vi "data_output_continuous.vi"() -> ()   [LabVIEW 2017]
uses:
  <vilib>/Utility/error.llb/DialogType.ctl
  <vilib>/DAQmx/write.llb/DAQmx Write (Analog 1D Wfm NChan NSamp).vi
  <vilib>/Utility/file.llb/Read Delimited Spreadsheet (DBL).vi
  <vilib>/DAQmx/create/channels.llb/DAQmx Create Channel (AO-Voltage-Basic).vi
  <vilib>/DAQmx/configure/timing.llb/DAQmx Timing (Sample Clock).vi
  <vilib>/DAQmx/miscellaneous.llb/DAQmx Fill In Error Info.vi
panel:
  in  "OK Button":bool
  out "Amplitude":dbl
  in  "Reduce Amplitude":bool
  in  "Sample Rate":dbl=1000.0
  in  "Sample Clock Source":tag="OnboardClock"
  in  "Max Voltage":dbl=5.0
  in  "Min Voltage":dbl=-5.0
  in  "Physical Channel(s)":tag="Dev1/ao0"
  in  "Stop":bool
  out "Number of Samples Written per Channel":dbl
  out "Waveform Graph":dynamicdata(graph)
  out "Matrix Cols":dbl
  out "Matrix Rows":dbl
  in  "csv Path":path
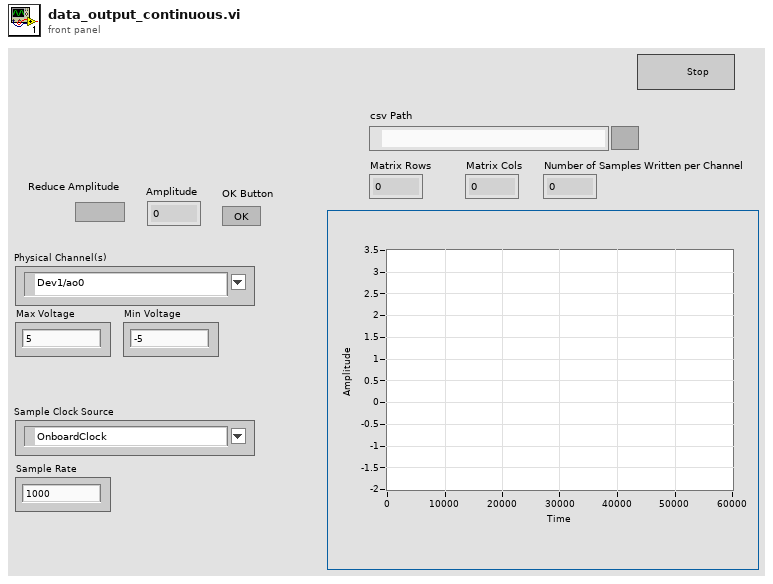
[diagram p1: front panel]
types:
  T1 = typedef "DialogType.ctl" = u16
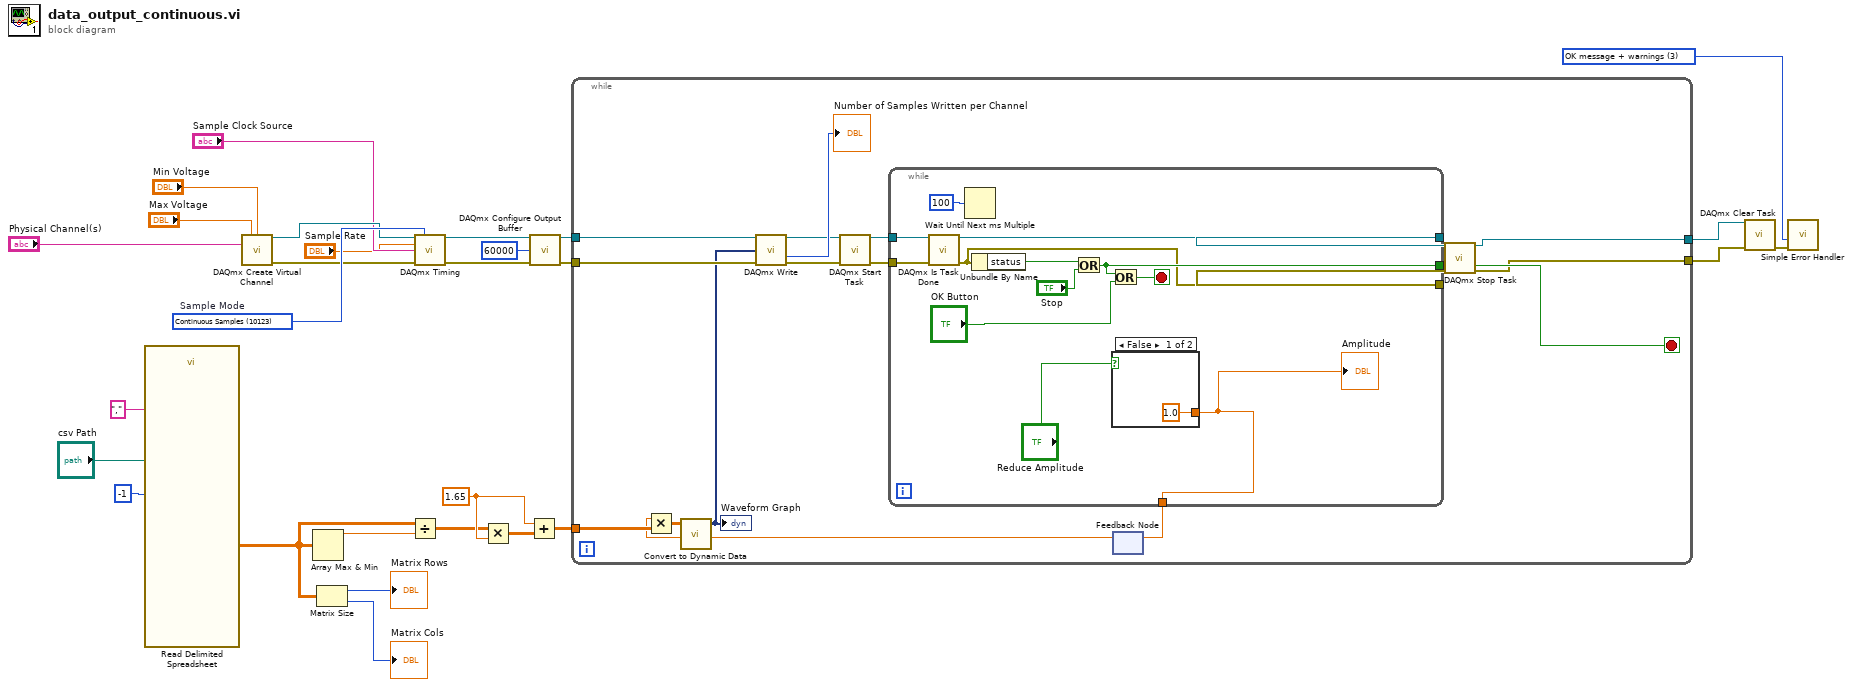
[diagram p0: block diagram]
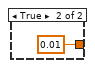
[diagram p2: hidden frame]
diagram:
  w17 = 10123 items=["Finite Samples"=10178, "Continuous Samples"=10123, "Hardware Timed Single Point"=12522]  # Sample Mode
  w18 = T1 3 items=["no dialog", "OK message", "continue or stop message", "OK message + warnings", "continue/stop + warnings"] ("type of dialog (OK msg:1)")
  w23 = 1.65
  n1 = call-poly <vilib>:"Read Delimited Spreadsheet.vi"("file path (dialog if empty)"="csv Path", "number of rows (all:-1)"=-1, "delimiter (\\t)"=",") -> ("all rows"=w3:dbl[][])  [unwired: 7 in, 5 out]
  n2 = call-poly <vilib>:"DAQmx Create Virtual Channel.vi"("maximum value"="Max Voltage", "minimum value"="Min Voltage", "physical channels"="Physical Channel(s)") -> ("task out"=w15:refnum<k21>, "error out"=w16:errorcluster)  [unwired: 11 in]
  n3 = Array Max & Min(array=w3) -> (max value=w25:dbl)  [unwired: 3 out]
  n4 = Matrix Size(0:w3) -> (1:→"Matrix Rows":i32, 2:→"Matrix Cols":i32)
  n5 = Divide(x=w3, y=w25) -> (x/y=w22:dbl[][])
  n6 = call-poly <vilib>:"DAQmx Timing.vi"("task/channels in"=w15, "sample mode"=w17, "rate"="Sample Rate", "source"="Sample Clock Source", "error in"=w16) -> ("task out"=w9:refnum<k21>, "error out"=w7:errorcluster)  [unwired: 9 in]
  n7 = Multiply(x=w22, y=w23) -> (x*y=w24:dbl[][])
  n8 = Add(x=w23, y=w24) -> (x+y=w4:dbl[][])
  n9 = call <vilib>:"DAQmx Configure Output Buffer.vi"("task/channels in"=w9, "buffer size (in samples per channel)"=60000, "error in"=w7) -> ("task out"=w6:refnum<k21>, "error out"=w5:errorcluster)  [unwired: 11 in]
  n10 = while {
    tunnel: w6 -> [w40]
    tunnel: w5 -> [w39]
    tunnel: w4 -> [w36]
    tunnel: [w31] -> w2
    tunnel: [w30] -> w1
    stop <- w37 stop-if-true
    n11 = feedback #1() -> (w34:dbl)  [unwired: 1 in]
    n12 = Multiply(x=w34, y=w36) -> (x*y=w35:dbl[][])
    n13 = call "Convert to Dynamic Data"("2D Array"=w35) -> ("Dynamic Data Type"=w38:dynamicdata)  [unwired: 3 in]
    "Waveform Graph" <- w38
    n14 = call-poly <vilib>:"DAQmx Write.vi"("task/channels in"=w40, "data"=w38, "error in"=w39) -> ("task out"=w44:refnum<k21>, "number of samples written per channel"=→"Number of Samples Written per Channel":u32, "error out"=w43:errorcluster)  [unwired: 10 in]
    n15 = call <vilib>:"DAQmx Start Task.vi"("task/channels in"=w44, "error in"=w43) -> ("task out"=w41:refnum<k21>, "error out"=w42:errorcluster)  [unwired: 12 in]
    n16 = while {
      tunnel: w41 -> [w54]
      tunnel: w42 -> [w53]
      tunnel: [w51] -> w37
      tunnel: [w50] -> w33
      tunnel: [w49] -> w32
      tunnel: [w46] -> w29
      stop <- w52 stop-if-true
      n17 = call <vilib>:"DAQmx Is Task Done.vi"("task/channels in"=w54, "error in"=w53) -> ("task out"=w50:refnum<k21>, "error out"=w49:errorcluster)  [unwired: 11 in, 1 out]
      n18 = Wait Until Next ms Multiple(millisecond multiple=u32 100) -> ()  [unwired: 1 out]
      n19 = Unbundle By Name(w49) -> ("status"=w57:bool)
      n20 = Or(x=w57, y="Stop") -> (x .or. y?=w51:bool)
      n21 = Or(x=w51, y="OK Button") -> (x .or. y?=w52:bool)
      n22 = case shown="False" "Reduce Amplitude" {
        tunnel: [1.0 0.01] -> w46
        frame False {
        }
        frame True {
        }
      }
      "Amplitude" <- w46
    }
    n23 = feedback-in #1(w29) -> ()
    n24 = call <vilib>:"DAQmx Stop Task.vi"("task/channels in"=w33, "error in"=w32) -> ("task out"=w31:refnum<k21>, "error out"=w30:errorcluster)  [unwired: 12 in]
  }
  n25 = call <vilib>:"DAQmx Clear Task.vi"("task in"=w2, "error in"=w1) -> ("error out"=w19:errorcluster)  [unwired: 13 in]
  n26 = call <vilib>:"Simple Error Handler.vi"("type of dialog (OK msg:1)"=w18, "error in (no error)"=w19) -> ()  [unwired: 3 in, 5 out]
